vi "BuildRelease_Interface_RunVI(2013-XXXX).vi"(8 "error in (no error)":errorcluster, 10 "VI of LvClass that implements this interface VI":refnum<vi>, 11 "Interface VI":refnum<vi>) -> (0 "error out":errorcluster, 3 "LvClassObjectDataOut(If the VI has a LVClass Indicator)":variant)   [LabVIEW 2013]
doc: "This implemetation is for LV2013 or later."
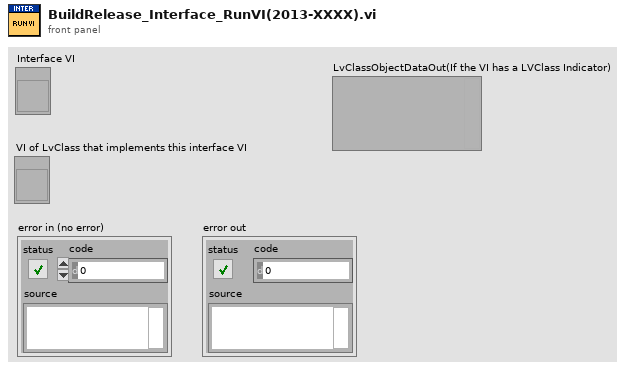
[diagram p1: front panel]
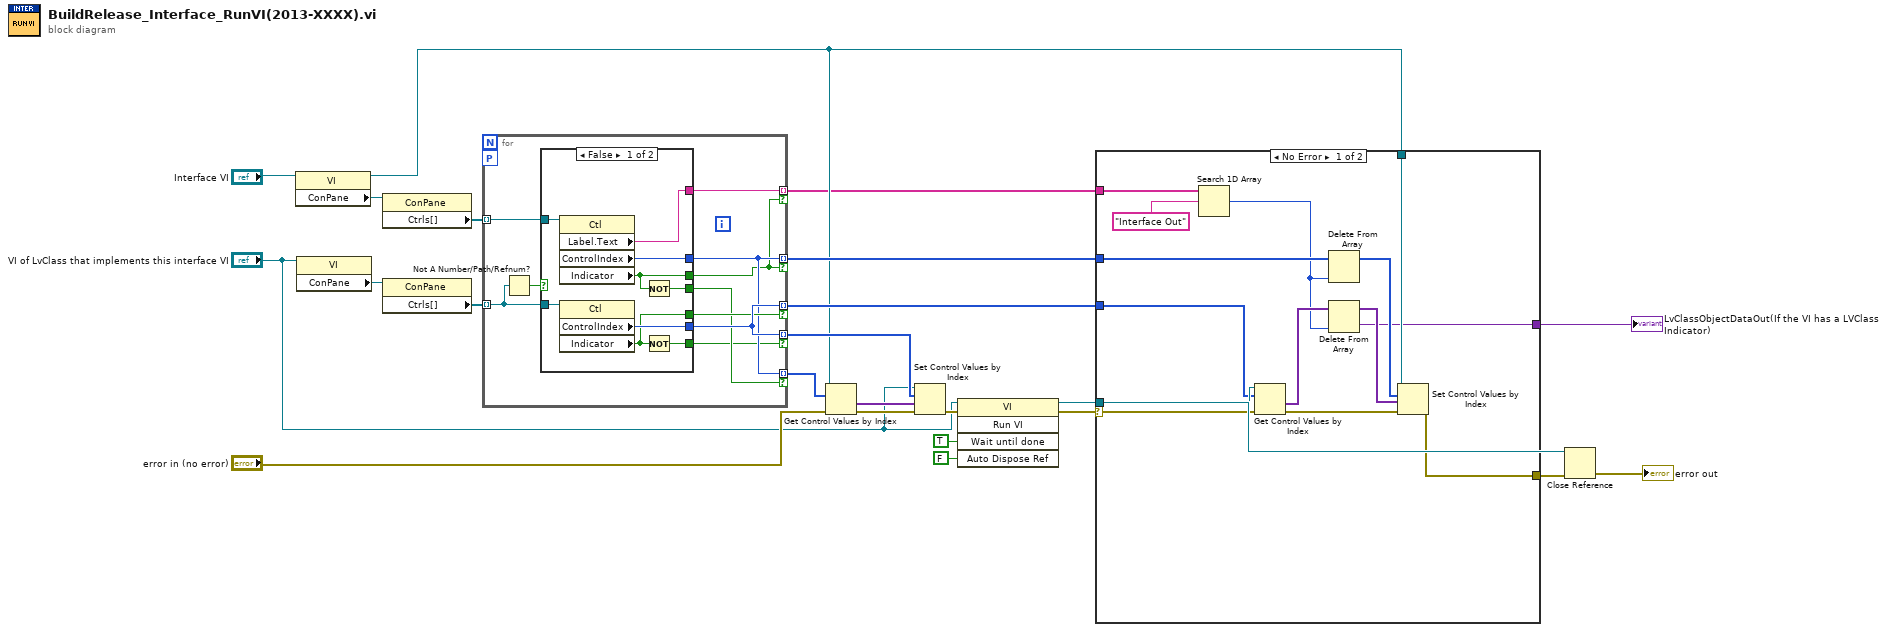
[diagram p0: block diagram]
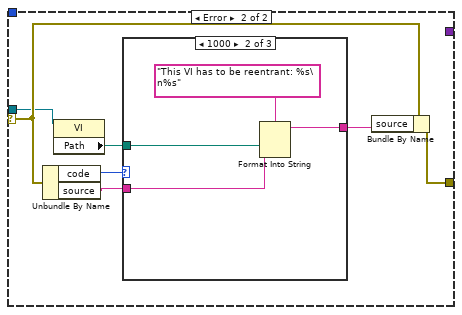
[diagram p2: hidden frame]
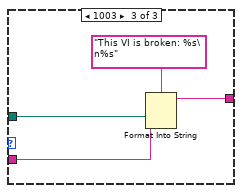
[diagram p4: hidden frame]
diagram:
  n1 = property class="VI"(reference="Interface VI") -> (reference out=w7:refnum<vi>, "ConPane"=w18:refnum<vi>)  [unwired: 1 in, 1 out]
  n2 = property class="VI"(reference="VI of LvClass that implements this interface VI") -> ("ConPane"=w20:refnum<vi>)  [unwired: 1 in, 2 out]
  n3 = property class="ConPane"(reference=w18) -> ("Ctrls[]"=w17:refnum<vi>[])  [unwired: 1 in, 2 out]
  n4 = property class="ConPane"(reference=w20) -> ("Ctrls[]"=w19:refnum<vi>[])  [unwired: 1 in, 2 out]
  n5 = for {
    tunnel: w19 -> [w32] mode=indexing
    tunnel: [w33] -> w21 mode=indexing if=w26
    tunnel: [w33] -> w8 mode=indexing if=w30
    tunnel: w17 -> [w29] mode=indexing
    tunnel: [w28] -> w16 mode=indexing if=w27
    tunnel: [w28] -> w13 mode=indexing if=w24
    tunnel: [w25] -> w1 mode=indexing if=w24
    workers-P: _ -> [_]
    n6 = Not A Number/Path/Refnum?(number/path/refnum=w32) -> (NaN/Path/Refnum?=w31:bool)
    n7 = case shown="False" w31 {
      tunnel: [w42 _] -> w33
      tunnel: [w36 _] -> w30
      tunnel: w32 -> [w41 _]
      tunnel: w29 -> [w40 _]
      tunnel: [w39 _] -> w28
      tunnel: [w38 _] -> w24
      tunnel: [w37 _] -> w27
      tunnel: [w35 _] -> w26
      tunnel: [w34 _] -> w25
      frame False {
        n8 = property class="Ctl"(reference=w40) -> ("Label.Text"=w34:string, "ControlIndex"=w39:i32, "Indicator"=w38:bool)  [unwired: 1 in, 2 out]
        n9 = property class="Ctl"(reference=w41) -> ("ControlIndex"=w42:i32, "Indicator"=w36:bool)  [unwired: 1 in, 2 out]
        n10 = Not(x=w38) -> (.not. x?=w37:bool)
        n11 = Not(x=w36) -> (.not. x?=w35:bool)
      }
      frame True {
      }
    }
  }
  n12 = Get Control Values by Index(0:w7, 1:w16, 3:"error in (no error)") -> (10:w15:variant[], 11:w14:errorcluster)
  n13 = Set Control Values by Index(0:"VI of LvClass that implements this interface VI", 1:w21, 2:w15, 3:w14) -> (11:w23:errorcluster)
  n14 = invoke class="VI" method="Run VI"(reference="VI of LvClass that implements this interface VI", error in=w23, "Wait until done"=TRUE ("Wait Until Done"), "Auto Dispose Ref"=FALSE ("Auto Dispose Reference")) -> (reference out=w12:refnum<vi>, error out=w22:errorcluster)  [unwired: 1 in, 3 out]
  n15 = case shown="No Error" w22 {
    selector: w22 -> [w56 w59]
    tunnel: w13 -> [w53 _]
    tunnel: w1 -> [w45 _]
    tunnel: w12 -> [w50 w57]
    tunnel: [w49 w58] -> w11
    tunnel: w8 -> [w48 _]
    tunnel: w7 -> [w47 _]
    tunnel: [w46 _] -> w6
    frame No Error {
      n16 = Search 1D Array(1D array=w45, element="Interface Out") -> (index of element=w43:i32)  [unwired: 1 in]
      n17 = Get Control Values by Index(0:w50, 1:w48, 3:w56) -> (10:w52:variant[], 11:w55:errorcluster)
      n18 = Delete From Array(array=w53, index=w43) -> (array with subset deleted=w54:i32[])  [unwired: 1 in, 1 out]
      n19 = Delete From Array(array=w52, index=w43) -> (deleted portion=w46:variant, array with subset deleted=w51:variant[])  [unwired: 1 in]
      n20 = Set Control Values by Index(0:w47, 1:w54, 2:w51, 3:w55) -> (11:w49:errorcluster)
    }
    frame Error {
      n21 = Unbundle By Name(w59) -> ("code"=w61:i32, "source"=w62:string)
      n22 = property class="VI"(reference=w57) -> ("Path"=w63:path)  [unwired: 1 in, 2 out]
      n23 = case shown="1000" w61 {
        tunnel: w62 -> [w64 w67 w71]
        tunnel: [w64 w66 w70] -> w60
        tunnel: w63 -> [_ w65 w69]
        frame 0, Default {
        }
        frame 1000 {
          n24 = Format Into String(format string="This VI has to be reentrant: %s\n%s" ("string"), w65, w67) -> (resulting string=w66:string)  [unwired: 2 in, 1 out]
        }
        frame 1003 {
          n25 = Format Into String(format string="This VI is broken: %s\n%s" ("string"), w69, w71) -> (resulting string=w70:string)  [unwired: 2 in, 1 out]
        }
      }
      n26 = Bundle By Name(cluster=w59, "source"=w60) -> (w58:errorcluster)
    }
  }
  "LvClassObjectDataOut(If the VI has a LVClass Indicator)" <- w6
  n27 = Close Reference(reference=w12, error in (no error)=w11) -> (error out=→"error out":errorcluster)
